vi "odometry_calc_test.vi"() -> ()   [LabVIEW 2014]
uses:
  Common/Odometry.ctl
  Common/TwistCovariance.ctl
  <vilib>/robotics/Kinematics/Quaternion.ctl
  <vilib>/robotics/TaimiOmni/TaimiOmni/TaimiOmniVelocity.ctl
  <vilib>/robotics/Kinematics/RotateX.vi
  <vilib>/robotics/Kinematics/RotateY.vi
  <vilib>/robotics/Kinematics/RotateZ.vi
  <vilib>/Analysis/baseanly.llb/A x B.vi
  <vilib>/Analysis/baseanly.llb/Real A x B.vi
  <vilib>/robotics/Kinematics/Rotation Matrix to Angle Vector.vi
  <vilib>/robotics/TaimiOmni/TaimiOmni/TaimiOmni.lvclass
  <vilib>/robotics/Kinematics/NI_Kinematics.lvlib
panel:
  out "quaternion":T1
  out "OmniDynamics out":T2
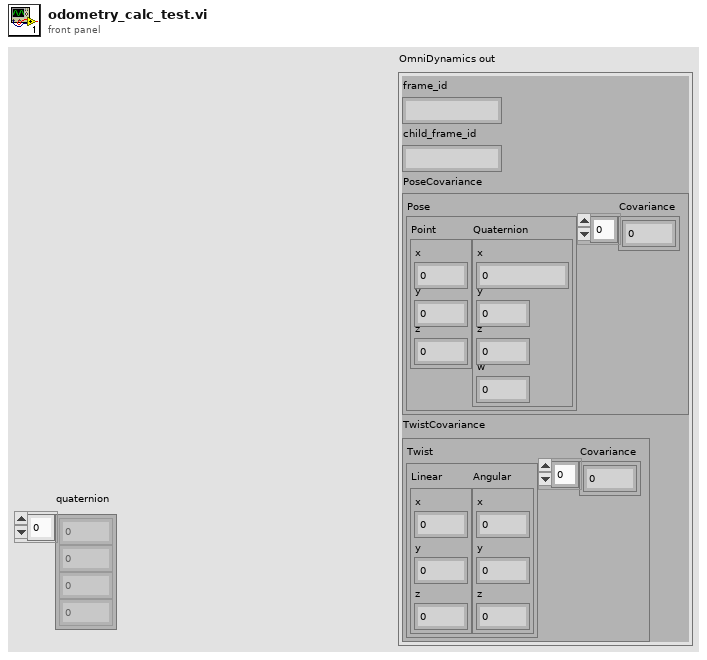
[diagram p1: front panel]
types:
  T1 = typedef "NI_Kinematics.lvlib/Quaternion.ctl" = dbl[]
  T2 = typedef "Odometry.ctl" = cluster{"frame_id":string, "child_frame_id":string, "PoseCovariance":cluster{"Pose":cluster{"Point":cluster{"x":dbl, "y":dbl, "z":dbl}, "Quaternion":cluster{"x":dbl, "y":dbl, "z":dbl, "w":dbl}}, "Covariance":dbl[]}, "TwistCovariance":T3}
  T3 = typedef "TwistCovariance.ctl" = cluster{"Twist":cluster{"Linear":cluster{"x":dbl, "y":dbl, "z":dbl}, "Angular":cluster{"x":dbl, "y":dbl, "z":dbl}}, "Covariance":dbl[]}
  T4 = typedef "TaimiOmni.lvclass/TaimiOmniVelocity.ctl" = cluster{"velX":dbl, "velY":dbl, "w":dbl}
  T5 = typedef "NI_Matrix.lvlib/RealMatrix.ctl" = dbl[][]
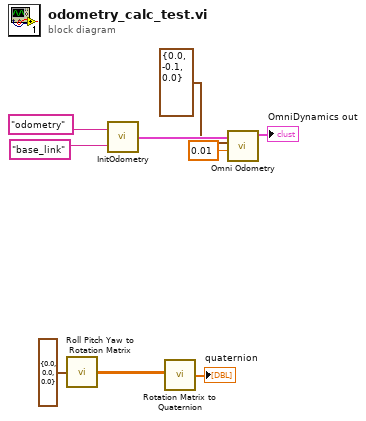
[diagram p0: block diagram]
diagram:
  n1 = call <vilib>:"Roll Pitch Yaw to Rotation Matrix.vi"("angles"=cluster{"roll":dbl, "pitch":dbl, "yaw":dbl} {"roll"=0.0, "pitch"=0.0, "yaw"=0.0}) -> ("rotation matrix"=w3:T5)
  n2 = call "InitOdometry.vi"("child_frame_id"="base_link" ("base_link"), "frame_id"="odometry" ("odometry_frame")) -> ("OmniDynamics out"=w7:T2)
  n3 = call <vilib>:"Rotation Matrix to Quaternion.vi"("rotation matrix"=w3) -> ("quaternion"=→"quaternion":T1)
  n4 = call "Omni Odometry.vi"("dt"=0.01, "TaimiOmniVelocity"=T4 {"velX"=0.0, "velY"=-0.1, "w"=0.0}, "OmniDynamics in"=w7) -> ("OmniDynamics out"=→"OmniDynamics out":T2)  [unwired: 8 in]
